vi "Default Search Path.vi"() -> (0 "Search Path":path[](array[path]))   [LabVIEW 2018, in "Toolkit.lvlib" / "Loaders.lvlib" / "File.lvclass"]
uses:
  File.lvclass
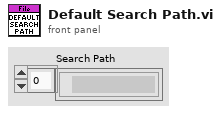
[diagram p1: front panel]
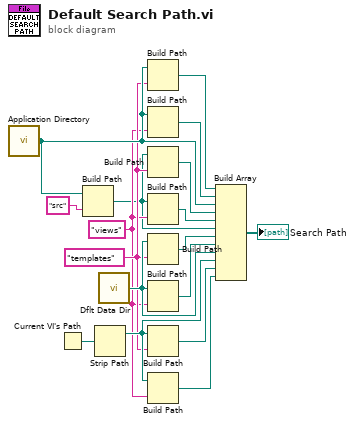
[diagram p0: block diagram]
diagram:
  w4 = "views" ("name or relative path")
  w5 = "templates" ("name or relative path")
  n1 = call <vilib>:"Application Directory.vi"() -> ("Application Directory"=w7:path)
  n2 = Current VI's Path() -> (path=w16:path)
  n3 = Build Path(base path=w7, name or relative path="src") -> (appended path=w1:path)
  n4 = Strip Path(path=w16) -> (stripped path=w10:path)  [unwired: 1 out]
  n5 = call <vilib>:"Dflt Data Dir.vi"() -> ("App:Default Data Directory"=w11:path)
  n6 = Build Path(base path=w7, name or relative path=w5) -> (appended path=w15:path)
  n7 = Build Path(base path=w7, name or relative path=w4) -> (appended path=w14:path)
  n8 = Build Path(base path=w1, name or relative path=w5) -> (appended path=w3:path)
  n9 = Build Path(base path=w1, name or relative path=w4) -> (appended path=w2:path)
  n10 = Build Path(base path=w11, name or relative path=w5) -> (appended path=w13:path)
  n11 = Build Path(base path=w11, name or relative path=w4) -> (appended path=w12:path)
  n12 = Build Path(base path=w10, name or relative path=w5) -> (appended path=w9:path)
  n13 = Build Path(base path=w10, name or relative path=w4) -> (appended path=w8:path)
  n14 = Build Array(w15, w14, w7, w3, w2, w1, w13, w12, w11, w10, w9, w8) -> (→"Search Path":path[])
